vi "GeoLookup.vi"(8 "Type":T2(ring), 11 "Data":T1) -> (3 "DataOut":T1)   [LabVIEW 2017]
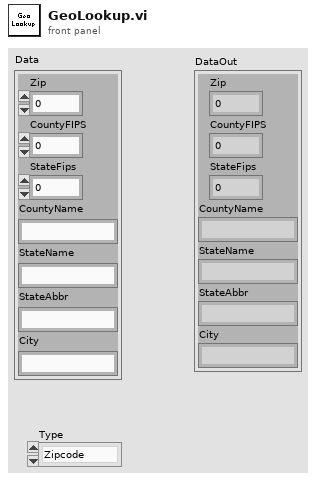
[diagram p1: front panel]
types:
  T1 = cluster{"Zip":i32, "CountyFIPS":i32, "StateFips":i32, "CountyName":string, "StateName":string, "StateAbbr":string, "City":string}
  T2 = enum16{"Zipcode", "CountyName", "StateName", "CountyFips", "StateFips", "StateAbbr", "CityState"}
  T3 = cluster{"Zip":i32[], "Fips":i32[], "StateFIPS":i32[], "City":string[], "County":string[], "State":string[], "StateName":string[], "EINS":i32[]}
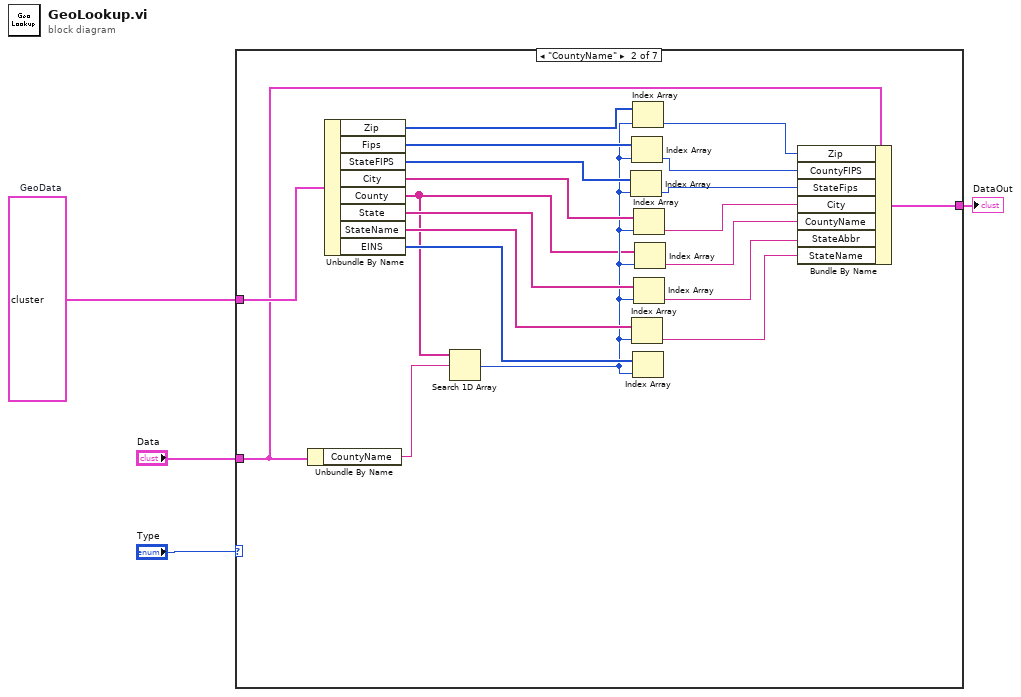
[diagram p0: block diagram]
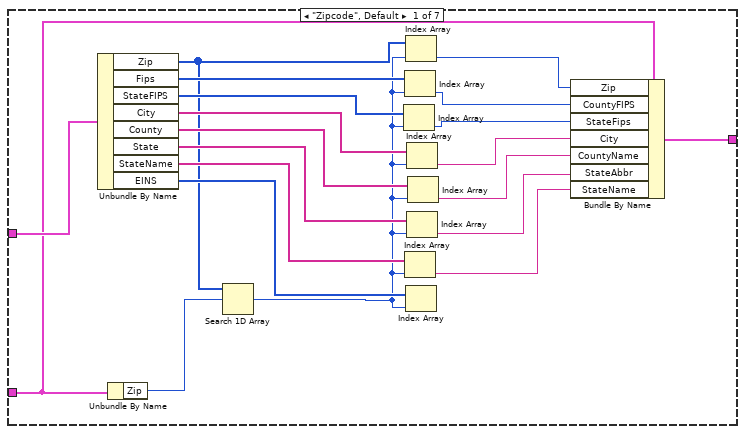
[diagram p2: hidden frame]
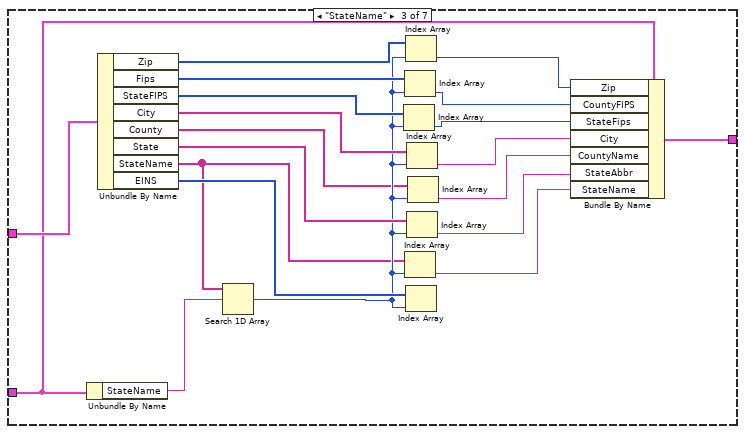
[diagram p3: hidden frame]
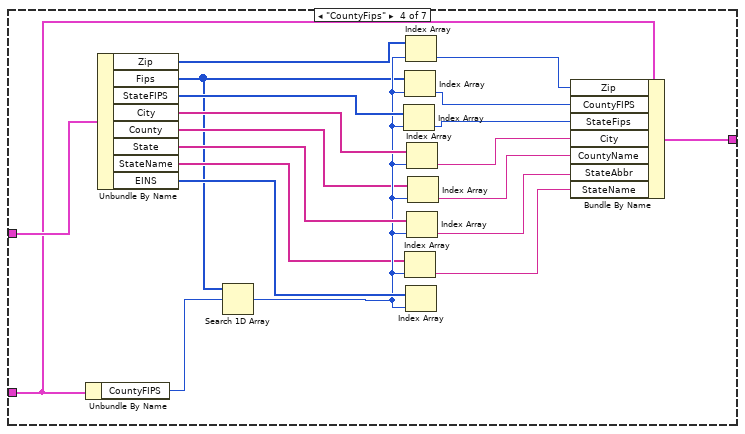
[diagram p4: hidden frame]
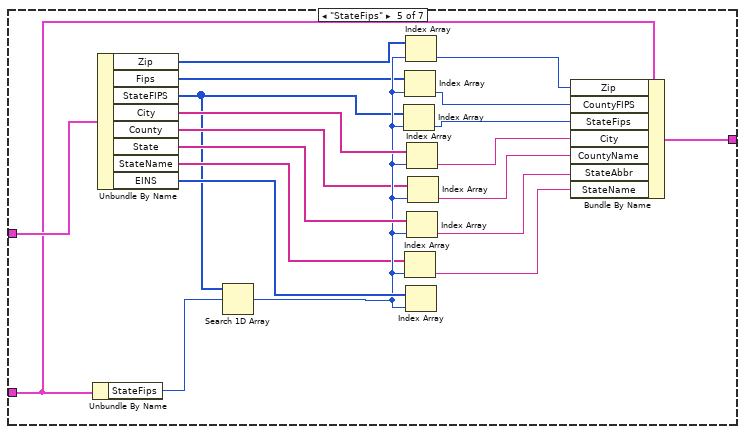
[diagram p5: hidden frame]
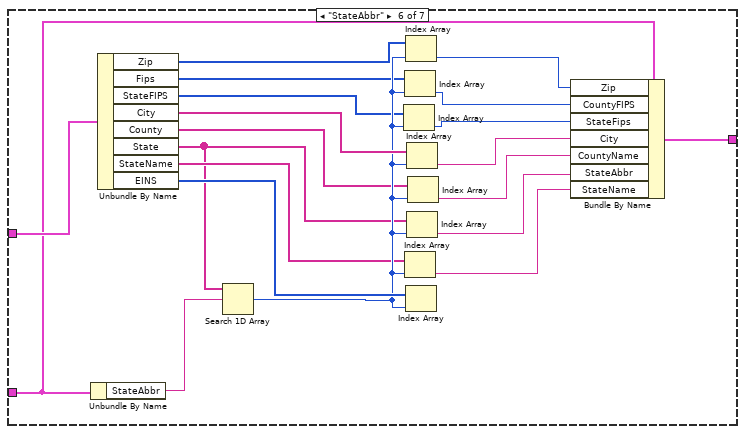
[diagram p6: hidden frame]
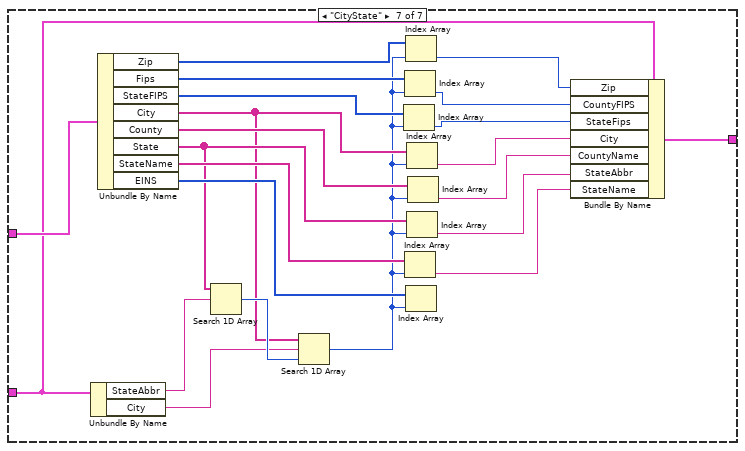
[diagram p7: hidden frame]
diagram:
  w2 = T3 {"Zip"=array[53962 elements], "Fips"=array[53962 elements], "StateFIPS"=array[53962 elements], "City"=array[53962 elements], "County"=array[53962 elements], "State"=array[53962 elements], "StateName"=array[53962 elements], "EINS"=array[53962 elements]}  # GeoData
  n1 = case shown="\"CountyName\"" "Type" {
    tunnel: "Data" -> [w12 w33 w54 w75 w96 w117 w141]
    tunnel: w2 -> [w16 w37 w58 w79 w100 w121 w144]
    tunnel: [w5 w26 w47 w68 w89 w110 w134] -> w1
    frame "Zipcode", Default {
      n2 = Unbundle By Name(w16) -> ("Zip"=w15:i32[], "Fips"=w23:i32[], "StateFIPS"=w22:i32[], "City"=w21:string[], "County"=w20:string[], "State"=w19:string[], "StateName"=w18:string[], "EINS"=w17:i32[])
      n3 = Unbundle By Name(w12) -> ("Zip"=w24:i32)
      n4 = Search 1D Array(1D array=w15, element=w24) -> (index of element=w14:i32)  [unwired: 1 in]
      n5 = Index Array(array=w22, index=w14) -> (element=w10:i32)
      n6 = Index Array(array=w23, index=w14) -> (element=w11:i32)
      n7 = Index Array(array=w18, index=w14) -> (element=w6:string)
      n8 = Index Array(array=w15, index=w14) -> (element=w13:i32)
      n9 = Index Array(array=w17, index=w14) -> ()  [unwired: 1 out]
      n10 = Index Array(array=w21, index=w14) -> (element=w9:string)
      n11 = Index Array(array=w19, index=w14) -> (element=w7:string)
      n12 = Index Array(array=w20, index=w14) -> (element=w8:string)
      n13 = Bundle By Name(cluster=w12, "Zip"=w13, "CountyFIPS"=w11, "StateFips"=w10, "City"=w9, "CountyName"=w8, "StateAbbr"=w7, "StateName"=w6) -> (w5:T1)
    }
    frame "CountyName" {
      n14 = Unbundle By Name(w33) -> ("CountyName"=w44:string)
      n15 = Unbundle By Name(w37) -> ("Zip"=w36:i32[], "Fips"=w43:i32[], "StateFIPS"=w42:i32[], "City"=w41:string[], "County"=w25:string[], "State"=w40:string[], "StateName"=w39:string[], "EINS"=w38:i32[])
      n16 = Search 1D Array(1D array=w25, element=w44) -> (index of element=w35:i32)  [unwired: 1 in]
      n17 = Index Array(array=w42, index=w35) -> (element=w31:i32)
      n18 = Index Array(array=w43, index=w35) -> (element=w32:i32)
      n19 = Index Array(array=w39, index=w35) -> (element=w27:string)
      n20 = Index Array(array=w36, index=w35) -> (element=w34:i32)
      n21 = Index Array(array=w38, index=w35) -> ()  [unwired: 1 out]
      n22 = Index Array(array=w41, index=w35) -> (element=w30:string)
      n23 = Index Array(array=w40, index=w35) -> (element=w28:string)
      n24 = Index Array(array=w25, index=w35) -> (element=w29:string)
      n25 = Bundle By Name(cluster=w33, "Zip"=w34, "CountyFIPS"=w32, "StateFips"=w31, "City"=w30, "CountyName"=w29, "StateAbbr"=w28, "StateName"=w27) -> (w26:T1)
    }
    frame "StateName" {
      n26 = Unbundle By Name(w54) -> ("StateName"=w64:string)
      n27 = Unbundle By Name(w58) -> ("Zip"=w57:i32[], "Fips"=w63:i32[], "StateFIPS"=w62:i32[], "City"=w61:string[], "County"=w46:string[], "State"=w60:string[], "StateName"=w45:string[], "EINS"=w59:i32[])
      n28 = Search 1D Array(1D array=w45, element=w64) -> (index of element=w56:i32)  [unwired: 1 in]
      n29 = Index Array(array=w62, index=w56) -> (element=w52:i32)
      n30 = Index Array(array=w63, index=w56) -> (element=w53:i32)
      n31 = Index Array(array=w45, index=w56) -> (element=w48:string)
      n32 = Index Array(array=w57, index=w56) -> (element=w55:i32)
      n33 = Index Array(array=w59, index=w56) -> ()  [unwired: 1 out]
      n34 = Index Array(array=w61, index=w56) -> (element=w51:string)
      n35 = Index Array(array=w60, index=w56) -> (element=w49:string)
      n36 = Index Array(array=w46, index=w56) -> (element=w50:string)
      n37 = Bundle By Name(cluster=w54, "Zip"=w55, "CountyFIPS"=w53, "StateFips"=w52, "City"=w51, "CountyName"=w50, "StateAbbr"=w49, "StateName"=w48) -> (w47:T1)
    }
    frame "CountyFips" {
      n38 = Unbundle By Name(w75) -> ("CountyFIPS"=w84:i32)
      n39 = Unbundle By Name(w79) -> ("Zip"=w78:i32[], "Fips"=w65:i32[], "StateFIPS"=w83:i32[], "City"=w82:string[], "County"=w67:string[], "State"=w81:string[], "StateName"=w66:string[], "EINS"=w80:i32[])
      n40 = Search 1D Array(1D array=w65, element=w84) -> (index of element=w77:i32)  [unwired: 1 in]
      n41 = Index Array(array=w83, index=w77) -> (element=w73:i32)
      n42 = Index Array(array=w65, index=w77) -> (element=w74:i32)
      n43 = Index Array(array=w66, index=w77) -> (element=w69:string)
      n44 = Index Array(array=w78, index=w77) -> (element=w76:i32)
      n45 = Index Array(array=w80, index=w77) -> ()  [unwired: 1 out]
      n46 = Index Array(array=w82, index=w77) -> (element=w72:string)
      n47 = Index Array(array=w81, index=w77) -> (element=w70:string)
      n48 = Index Array(array=w67, index=w77) -> (element=w71:string)
      n49 = Bundle By Name(cluster=w75, "Zip"=w76, "CountyFIPS"=w74, "StateFips"=w73, "City"=w72, "CountyName"=w71, "StateAbbr"=w70, "StateName"=w69) -> (w68:T1)
    }
    frame "StateFips" {
      n50 = Unbundle By Name(w96) -> ("StateFips"=w104:i32)
      n51 = Unbundle By Name(w100) -> ("Zip"=w99:i32[], "Fips"=w86:i32[], "StateFIPS"=w85:i32[], "City"=w103:string[], "County"=w88:string[], "State"=w102:string[], "StateName"=w87:string[], "EINS"=w101:i32[])
      n52 = Search 1D Array(1D array=w85, element=w104) -> (index of element=w98:i32)  [unwired: 1 in]
      n53 = Index Array(array=w85, index=w98) -> (element=w94:i32)
      n54 = Index Array(array=w86, index=w98) -> (element=w95:i32)
      n55 = Index Array(array=w87, index=w98) -> (element=w90:string)
      n56 = Index Array(array=w99, index=w98) -> (element=w97:i32)
      n57 = Index Array(array=w101, index=w98) -> ()  [unwired: 1 out]
      n58 = Index Array(array=w103, index=w98) -> (element=w93:string)
      n59 = Index Array(array=w102, index=w98) -> (element=w91:string)
      n60 = Index Array(array=w88, index=w98) -> (element=w92:string)
      n61 = Bundle By Name(cluster=w96, "Zip"=w97, "CountyFIPS"=w95, "StateFips"=w94, "City"=w93, "CountyName"=w92, "StateAbbr"=w91, "StateName"=w90) -> (w89:T1)
    }
    frame "StateAbbr" {
      n62 = Unbundle By Name(w117) -> ("StateAbbr"=w124:string)
      n63 = Unbundle By Name(w121) -> ("Zip"=w120:i32[], "Fips"=w107:i32[], "StateFIPS"=w106:i32[], "City"=w123:string[], "County"=w109:string[], "State"=w105:string[], "StateName"=w108:string[], "EINS"=w122:i32[])
      n64 = Search 1D Array(1D array=w105, element=w124) -> (index of element=w119:i32)  [unwired: 1 in]
      n65 = Index Array(array=w106, index=w119) -> (element=w115:i32)
      n66 = Index Array(array=w107, index=w119) -> (element=w116:i32)
      n67 = Index Array(array=w108, index=w119) -> (element=w111:string)
      n68 = Index Array(array=w120, index=w119) -> (element=w118:i32)
      n69 = Index Array(array=w122, index=w119) -> ()  [unwired: 1 out]
      n70 = Index Array(array=w123, index=w119) -> (element=w114:string)
      n71 = Index Array(array=w105, index=w119) -> (element=w112:string)
      n72 = Index Array(array=w109, index=w119) -> (element=w113:string)
      n73 = Bundle By Name(cluster=w117, "Zip"=w118, "CountyFIPS"=w116, "StateFips"=w115, "City"=w114, "CountyName"=w113, "StateAbbr"=w112, "StateName"=w111) -> (w110:T1)
    }
    frame "CityState" {
      n74 = Unbundle By Name(w141) -> ("StateAbbr"=w146:string, "City"=w126:string)
      n75 = Unbundle By Name(w144) -> ("Zip"=w143:i32[], "Fips"=w131:i32[], "StateFIPS"=w130:i32[], "City"=w127:string[], "County"=w133:string[], "State"=w129:string[], "StateName"=w132:string[], "EINS"=w145:i32[])
      n76 = Search 1D Array(1D array=w129, element=w146) -> (index of element=w128:i32)  [unwired: 1 in]
      n77 = Search 1D Array(1D array=w127, element=w126, start index (0)=w128) -> (index of element=w125:i32)
      n78 = Index Array(array=w130, index=w125) -> (element=w139:i32)
      n79 = Index Array(array=w131, index=w125) -> (element=w140:i32)
      n80 = Index Array(array=w132, index=w125) -> (element=w135:string)
      n81 = Index Array(array=w143, index=w125) -> (element=w142:i32)
      n82 = Index Array(array=w145, index=w125) -> ()  [unwired: 1 out]
      n83 = Index Array(array=w127, index=w125) -> (element=w138:string)
      n84 = Index Array(array=w129, index=w125) -> (element=w136:string)
      n85 = Index Array(array=w133, index=w125) -> (element=w137:string)
      n86 = Bundle By Name(cluster=w141, "Zip"=w142, "CountyFIPS"=w140, "StateFips"=w139, "City"=w138, "CountyName"=w137, "StateAbbr"=w136, "StateName"=w135) -> (w134:T1)
    }
  }
  "DataOut" <- w1
